vi "DHE_SetNPixSamples.vi"(7 "Database RefNum in":T1, 8 "error in (no error)":errorcluster, 9 "check sampling":bool=TRUE, 10 "nsamples":i32, 11 "fd":i32) -> (0 "error IO":errorcluster, 1 "DHE_OBS":T2 {"exptime" format="%.2f"}, 2 "return value":i32, 3 "fd out":i32)   [LabVIEW 2016]
uses:
  DHE_Obs.ctl
  DBSHAND/private/vis/DatabaseHand_RefNum.ctl
  DBSHAND/private/vis/DatabaseHand_Element_Get(string).vi
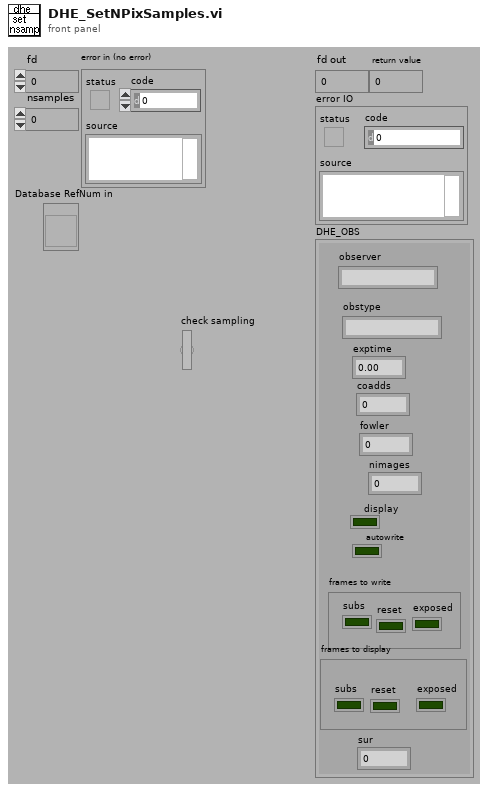
[diagram p1: front panel]
types:
  T1 = typedef "DatabaseHand_RefNum.ctl" = refnum<vi>
  T2 = typedef "DHE_Obs.ctl" = cluster{"observer":string, "obstype":string, "exptime":dbl, "coadds":i32, "fowler":i32, "nimages":i32, "display":bool, "autowrite":bool, "frames to write":cluster{"subs":bool, "reset":bool, "exposed":bool}, "frames to display":cluster{"subs":bool, "reset":bool, "exposed":bool}, "sur":i32}
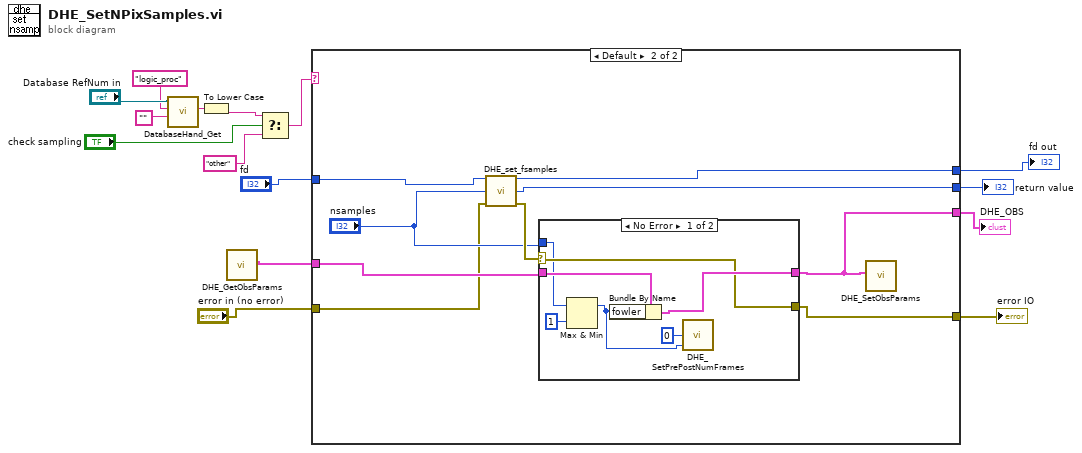
[diagram p0: block diagram]
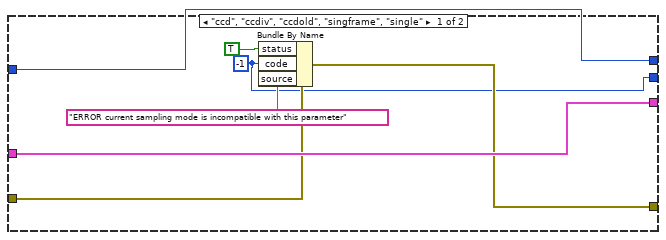
[diagram p2: hidden frame]
diagram:
  n1 = call-poly "DatabaseHand_Get.vi"("default value"="", "name"="logic_proc", "Database RefNum in"="Database RefNum in") -> ("value"=w8:string)  [unwired: 2 in, 6 out]
  n2 = To Lower Case(string=w8) -> (all lower case string=w3:string)
  n3 = call "DHE_GetObsParams.vi"() -> ("DHE_OBS"=w11:T2)  [unwired: 11 out]
  n4 = Select(t=w3, s="check sampling", f="other") -> (s? t:f=w2:string)
  n5 = case shown="Default" w2 {
    tunnel: [w22 w29] -> w12
    tunnel: w11 -> [w22 w28]
    tunnel: "error in (no error)" -> [w21 w27]
    tunnel: [w19 w26] -> w9
    tunnel: "fd" -> [w16 w25]
    tunnel: [w16 w24] -> w6
    tunnel: [w17 w23] -> w5
    frame "ccd", "ccdiv", "ccdold", "singframe", "single" {
      w17 = -1 ("code")
      n6 = Bundle By Name(cluster=w21, "status"=TRUE, "code"=w17, "source"="ERROR current sampling mode is incompatible with this parameter") -> (w19:errorcluster)
    }
    frame Default {
      n7 = call "DHE_set_fsamples.vi"("fd"=w25, "val"="nsamples", "error in (no error)"=w27) -> ("fd out"=w24:i32, "return value"=w23:i32, "error out"=w31:errorcluster)  [unwired: 10 out]
      n8 = case shown="No Error" w31 {
        selector: w31 -> [w36 w39]
        tunnel: "nsamples" -> [w34 _]
        tunnel: w28 -> [w38 w40]
        tunnel: [w37 w40] -> w29
        tunnel: [w36 w39] -> w26
        frame No Error {
          n9 = Max & Min(x=w34, y=1) -> (max(x,y)=w33:i32)  [unwired: 1 out]
          n10 = Bundle By Name(cluster=w38, "fowler"=w33) -> (w37:T2)
          n11 = call "DHE_SetPrePostNumFrames.vi"("DHE_PreExpose"=0, "DHE_PostExpose"=w33) -> ()  [unwired: 8 out]
        }
        frame Error {
        }
      }
      n12 = call "DHE_SetObsParams.vi"("DHE_OBS"=w29) -> ()  [unwired: 11 out]
    }
  }
  "DHE_OBS" <- w12
  "error IO" <- w9
  "fd out" <- w6
  "return value" <- w5
